vi "Do.vi"(8 "error in (no error)":errorcluster, 10 "Actor in":refnum<class "Actor.lvclass">, 11 "Prompt User for File Path to Load From":refnum<class "Prompt User for File Path to Load From.lvclass">) -> (0 "error out":errorcluster, 2 "Actor out":refnum<class "Actor.lvclass">)   [LabVIEW 2015, in "Measurement UI.lvlib" / "Prompt User for File Path to Load From.lvclass"]
uses:
  Prompt User for File Path to Load From.lvclass
  <vilib>/ActorFramework/Actor/Actor.lvclass
  Measurement UI.lvclass
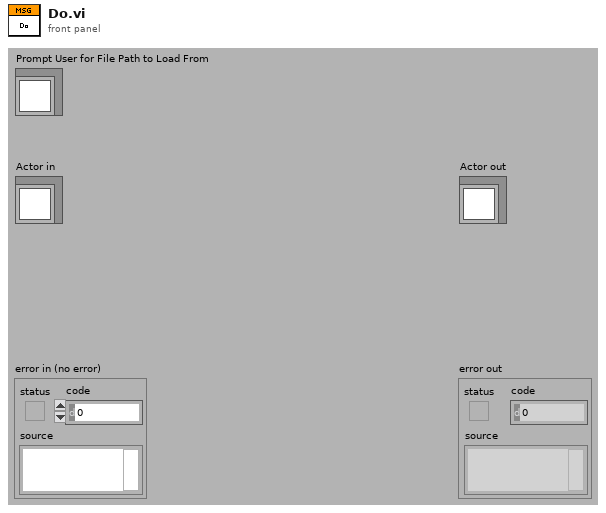
[diagram p1: front panel]
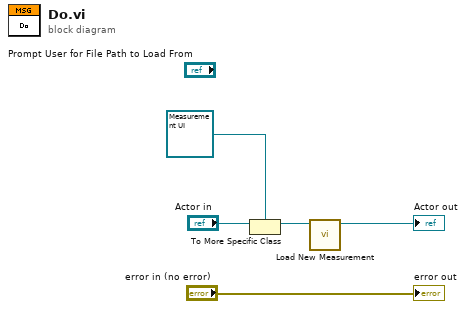
[diagram p0: block diagram]
diagram:
  n1 = To More Specific Class(target class=refnum<class "Measurement UI.lvclass"> refnum ("UI.lvclass"), reference="Actor in") -> (specific class reference=w2:refnum<class "Measurement UI.lvclass">)  [unwired: 1 in, 1 out]
  n2 = call-dynamic "Load New Measurement.vi"("UI in"=w2) -> ("UI out"=→"Actor out":refnum<class "Measurement UI.lvclass">)  [unwired: 9 in, 1 out]
  "error out" <- "error in (no error)"
